vi "简单运算.vi"() -> ()   [LabVIEW 2009]
panel:
  out "温度计":dbl(slide) scale=0.0..100.0 scale format="%#.2f"
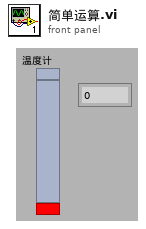
[diagram p1: front panel]
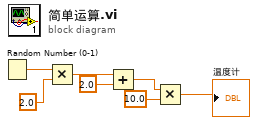
[diagram p0: block diagram]
diagram:
  n1 = Random Number (0-1)() -> (number: 0 to 1=w7:dbl)
  n2 = Multiply(x=w7, y=2.0) -> (x*y=w5:dbl)
  n3 = Add(x=w5, y=2.0) -> (x+y=w3:dbl)
  n4 = Multiply(x=w3, y=10.0) -> (x*y=→"温度计":dbl)
